vi "SubVI Tester.vi"() -> ()   [LabVIEW 2014]
uses:
  Weather Data.ctl
panel:
  out "Weather Data Out":T1={"Current Temperature"=0.0, "Max Temperature"=0.0, "Min Temperature"=0.0, "Temperature Warning?"=FALSE, "Temperature Warning Text"="No Warning", "Units"=0} {"Units" items=["Celsius", "Fahrenheit"]}
  in  "Min Temperature":dbl=10.0
  in  "Max Temperature":dbl=30.0
  in  "Stop":bool
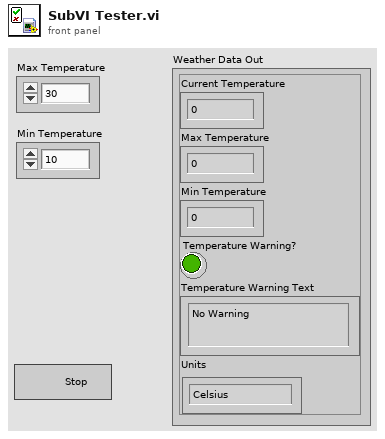
[diagram p1: front panel]
types:
  T1 = typedef "Weather Data.ctl" = cluster{"Current Temperature":dbl, "Max Temperature":dbl, "Min Temperature":dbl, "Temperature Warning?":bool, "Temperature Warning Text":string, "Units":u16}
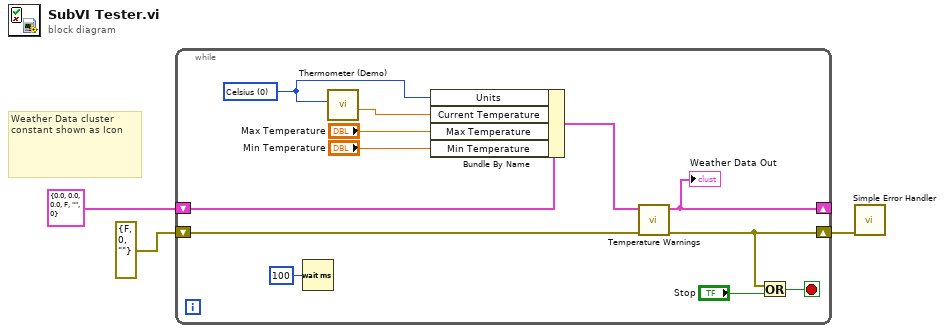
[diagram p0: block diagram]
diagram:
  # "Weather Data cluster constant shown as Icon"
  n1 = while {
    shift-right: [w6] -> _
    shift-left: T1 {"Current Temperature"=0.0, "Max Temperature"=0.0, "Min Temperature"=0.0, "Temperature Warning?"=FALSE, "Temperature Warning Text"="", "Units"=0} ("Weather Data In") -> [w15]
    shift-right: [w5] -> w2
    shift-left: errorcluster {"status"=FALSE, "code"=0, "source"=""} ("error out") -> [w11]
    stop <- w12 stop-if-true
    w4 = u16 0 items=["Celsius", "Fahrenheit"] ("Units (0: Celsius)")
    n2 = Wait (ms)(milliseconds to wait=u32 100) -> ()  [unwired: 1 out]
    n3 = call "Thermometer (Demo).vi"("Units (0: Celsius)"=w4) -> ("Temperature Value"=w7:dbl)  [unwired: 10 in]
    n4 = Bundle By Name(cluster=w15, "Units"=w4, "Current Temperature"=w7, "Max Temperature"="Max Temperature", "Min Temperature"="Min Temperature") -> (w10:T1)
    n5 = call "Temperature Warnings.vi"("Error In"=w11, "Weather Data In"=w10) -> ("Error Out"=w5:errorcluster, "Weather Data Out"=w6:T1)  [unwired: 8 in]
    "Weather Data Out" <- w6
    n6 = Or(x=w5, y="Stop") -> (x .or. y?=w12:bool)
  }
  n7 = call <vilib>:"Simple Error Handler.vi"("error in (no error)"=w2) -> ()  [unwired: 4 in, 5 out]
